vi "Lint.vi"() -> ()   [LabVIEW 2018, in "Scripts.lvlib"]
uses:
  Scripts.lvlib
  <vilib>/Field R&D Services/Labricator/Toolkit/Labricator.lvlib
panel:
  out "Tree":string(tree)
  # "Overview: Checks all Public VIs and Controls have VI documentation and their inputs and outputs have descriptions\nRequirements: LabVIEW, Labstache\nInstructions: Run this VI."
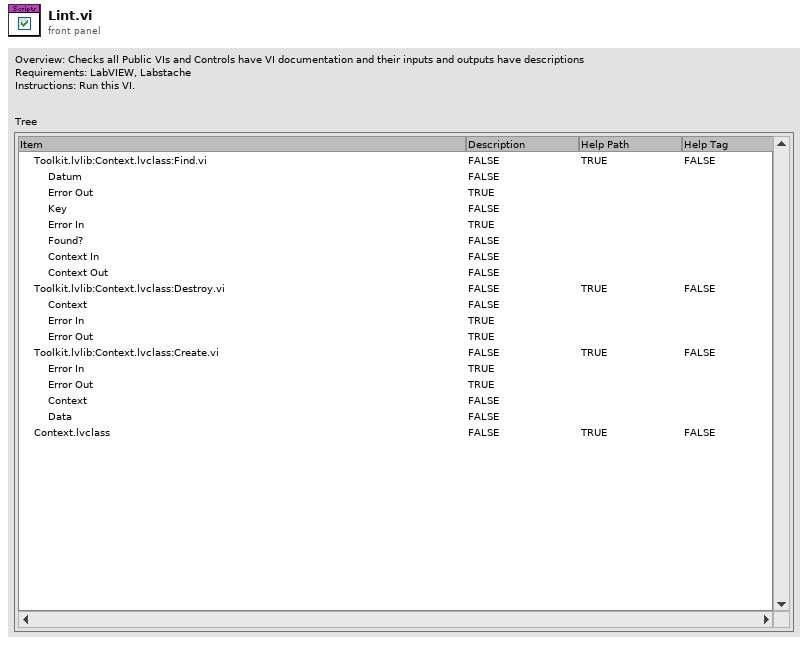
[diagram p1: front panel]
types:
  T1 = typedef "Scripts.lvlib/Project Item Lint Result.ctl" = cluster{"Description":bool, "Help Path":bool, "Help Tag":bool, "Project Item Name":string, "VI Controls":T2[]}
  T2 = typedef "Scripts.lvlib/VI Control Lint Result.ctl" = cluster{"Description":bool, "Name":string}
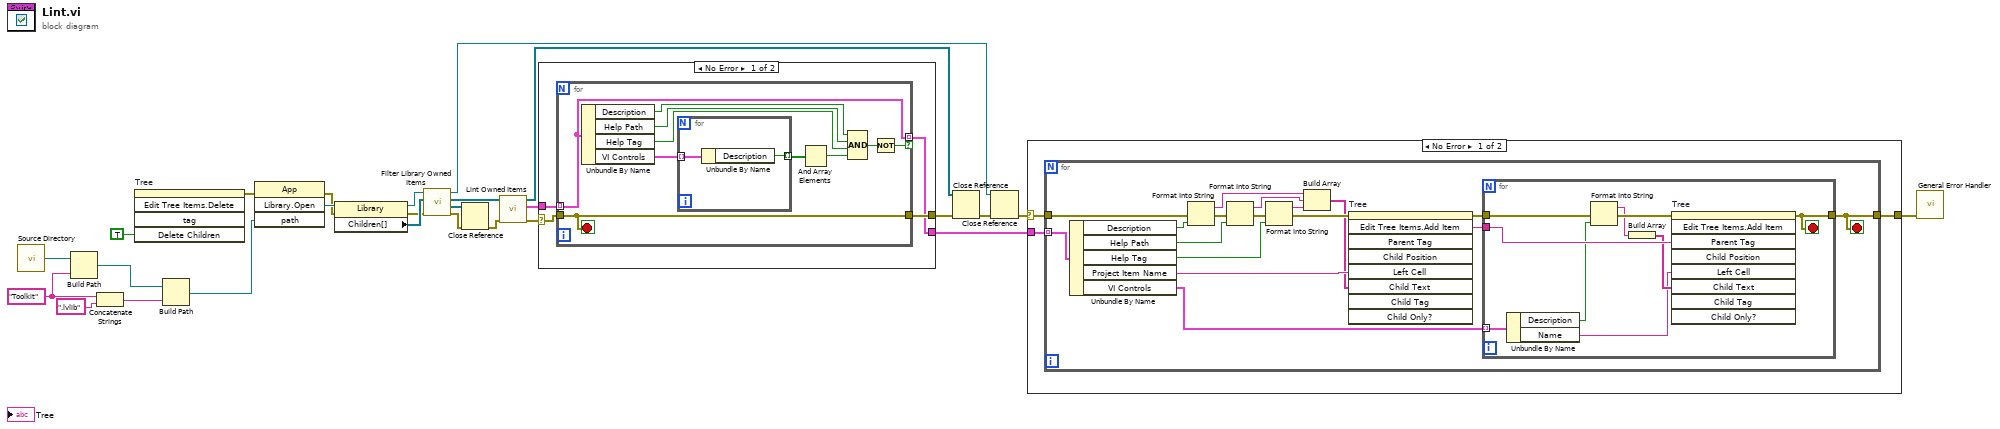
[diagram p0: block diagram]
diagram:
  w22 = "Toolkit" ("name or relative path")
  n1 = call <vilib>:"Source Directory.vi"() -> ("Source Directory"=w26:path)
  n2 = Build Path(base path=w26, name or relative path=w22) -> (appended path=w23:path)
  n3 = Concatenate Strings(w22, ".lvlib" ("string")) -> (w20:string)
  n4 = invoke on="Tree" class="Tree (strict)" method="Edit Tree Items.Delete"("Delete Children"=TRUE ("Delete Children?")) -> (error out=w1:errorcluster)  [unwired: 4 in, 4 out]
  n5 = Build Path(base path=w23, name or relative path=w20) -> (appended path=w19:path)
  n6 = invoke class="App" method="Library.Open"(error in=w1, "path"=w19) -> (error out=w9:errorcluster, "Open Library"=w24:refnum<vi>)  [unwired: 2 in, 2 out]
  n7 = property class="Library"(reference=w24, error in=w9) -> (reference out=w10:refnum<vi>, error out=w7:errorcluster, "Children[]"=w8:refnum<vi>[])
  n8 = call "Filter Library Owned Items.vi"("Error In"=w7, "Children[]"=w8, "Library Project Item In"=w10) -> ("Error Out"=w17:errorcluster, "Private Owned Items"=w16:refnum<vi>[], "Non-Private Owned Items"=w14:refnum<vi>[], "Library Project Item Out"=w18:refnum<vi>)  [unwired: 5 in]
  n9 = Close Reference(reference=w16, error in (no error)=w17) -> (error out=w15:errorcluster)
  n10 = call "Lint Owned Items.vi"("Error In"=w15, "Owned Items In"=w14) -> ("Error Out"=w4:errorcluster, "Results"=w12:T1[], "Owned Items Out"=w13:refnum<vi>[])  [unwired: 7 in]
  n11 = case shown="No Error" w4 {
    selector: w4 -> [w27 w43]
    tunnel: w12 -> [w30 _]
    tunnel: [w29 w43] -> w11
    tunnel: [w28 _] -> w5
    frame No Error {
      n12 = for {
        tunnel: w30 -> [w31] mode=indexing
        tunnel: [w31] -> w28 mode=indexing if=w35
        tunnel: w27 -> [w36]
        tunnel: [w36] -> w29
        stop <- w36 stop-if-true
        n13 = Unbundle By Name(w31) -> ("Description"=w40:bool, "Help Path"=w39:bool, "Help Tag"=w38:bool, "VI Controls"=w34:T2[])
        n14 = for {
          tunnel: w34 -> [w42] mode=indexing
          tunnel: [w41] -> w33 mode=indexing
          n15 = Unbundle By Name(w42) -> ("Description"=w41:bool)
        }
        n16 = And Array Elements(Boolean array=w33) -> (logical AND=w32:bool)
        n17 = Compound Arithmetic op=AND(w40, w39, w38, w32) -> (w37:bool)
        n18 = Not(x=w37) -> (.not. x?=w35:bool)
      }
    }
    frame Error {
    }
  }
  n19 = Close Reference(reference=w13, error in (no error)=w11) -> (error out=w25:errorcluster)
  n20 = Close Reference(reference=w18, error in (no error)=w25) -> (error out=w3:errorcluster)
  n21 = case shown="No Error" w3 {
    selector: w3 -> [w44 w73]
    tunnel: [w46 w73] -> w6
    tunnel: w5 -> [w45 _]
    frame No Error {
      n22 = for {
        tunnel: w45 -> [w63] mode=indexing
        tunnel: w44 -> [w61]
        tunnel: [w47] -> w46
        stop <- w47 stop-if-true
        n23 = Unbundle By Name(w63) -> ("Description"=w60:bool, "Help Path"=w56:bool, "Help Tag"=w55:bool, "Project Item Name"=w62:string, "VI Controls"=w48:T2[])
        n24 = Format Into String(error in=w61, w60) -> (resulting string=w54:string, error out=w59:errorcluster)  [unwired: 2 in]
        n25 = Format Into String(error in=w59, w56) -> (resulting string=w53:string, error out=w58:errorcluster)  [unwired: 2 in]
        n26 = Format Into String(error in=w58, w55) -> (resulting string=w52:string, error out=w57:errorcluster)  [unwired: 2 in]
        n27 = Build Array(w54, w53, w52) -> (w51:string[])
        n28 = invoke on="Tree" class="Tree (strict)" method="Edit Tree Items.Add Item"(error in=w57, "Left Cell"=w62, "Child Text"=w51) -> (error out=w50:errorcluster, "Edit Tree Items:Add Item"=w49:string)  [unwired: 6 in, 7 out]
        n29 = for {
          tunnel: w49 -> [w71]
          tunnel: w48 -> [w70] mode=indexing
          tunnel: w50 -> [w72]
          tunnel: [w64] -> w47
          stop <- w64 stop-if-true
          n30 = Unbundle By Name(w70) -> ("Description"=w68:bool, "Name"=w65:string)
          n31 = Format Into String(error in=w72, w68) -> (resulting string=w67:string, error out=w69:errorcluster)  [unwired: 2 in]
          n32 = Build Array(w67) -> (w66:string[])
          n33 = invoke on="Tree" class="Tree (strict)" method="Edit Tree Items.Add Item"(error in=w69, "Parent Tag"=w71, "Left Cell"=w65, "Child Text"=w66) -> (error out=w64:errorcluster)  [unwired: 5 in, 8 out]
        }
      }
    }
    frame Error {
    }
  }
  n34 = call <vilib>:"General Error Handler.vi"("error in (no error)"=w6) -> ()  [unwired: 10 in, 5 out]
